vi "Zamojski_Target_C_1.vi"() -> ()   [LabVIEW 2020]
uses:
  <vilib>/Platform/TimedLoop/XDataNode/timing_clust.ctl
  <vilib>/Platform/TimedLoop/XDataNode/nitl_modes.ctl
  <vilib>/Platform/TimedLoop/XDataNode/wakeup.ctl
  <vilib>/platform/TimedLoop/XDataNode/XDataNode.xnode
  <vilib>/Platform/TimedLoop/XDataNode/XDNodeRunTimeDep.lvlib
panel:
  out "timed out?":bool
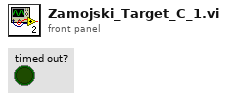
[diagram p1: front panel]
types:
  T1 = typedef "XDNodeRunTimeDep.lvlib/timing_clust.ctl" = cluster{"Expected End [f-1]":u64, "Actual End [f-1]":u64, "Finished Late? [f-1]":bool, "Expected End [i-1]":u64, "Actual End [i-1]":u64, "Finished Late? [i-1]":bool, "Expected Start [i]":u64, "Actual Start [i]":u64, "Expected Start [f]":u64, "Actual Start [f]":u64, "Source Name":string, "Structure Name":string, "Period":i64, "Deadline":i64, "Offset":i64, "Start":i64, "Priority":i32, "Timeout":i32, "Mode":T2, "Wakeup Reason":T3, "Error":errorcluster, "Source Type":string, "Secondary Source Type":string, "Global End Time":u64, "Global Start Time":u64, "Frame Duration":u64, "Iteration Duration":u64, "Assigned CPU":i32, "I/O Scan Engine Mode":u32}
  T2 = typedef "XDNodeRunTimeDep.lvlib/nitl_modes.ctl" = enum32{"No Change", "Process missed periods, maintain original phase", "Discard missed periods, maintain original phase", "Process missed periods, ignore original phase", "Discard missed periods, ignore original phase"}
  T3 = typedef "XDNodeRunTimeDep.lvlib/wakeup.ctl" = enum32{"Normal", "Aborted", "Asynchronous wakeup", "Timing source error", "Timed loop error", "Timeout"}
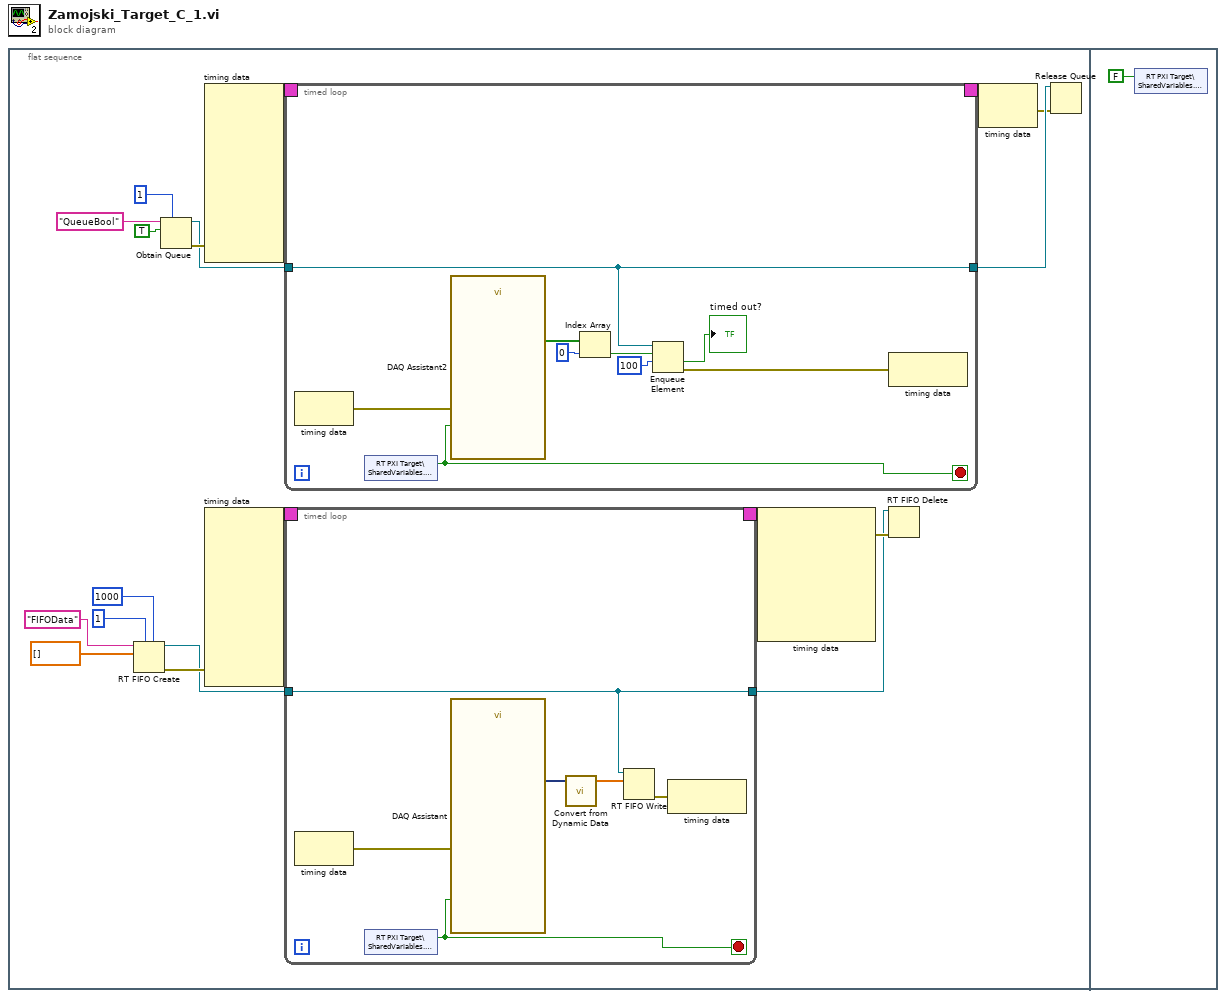
[diagram p0: block diagram]
diagram:
  n1 = flat-sequence {
    frame #0 {
      n2 = RT FIFO Create(0:"FIFOData" ("name (unnamed)"), 1:dbl[] [], 4:u32 1 ("size (10)"), 6:u32 1000 ("elements in array (1)")) -> (8:w11:refnum<k33>, 11:w15:errorcluster)  [unwired: 4 in, 1 out]
      n3 = Obtain Queue(max queue size (-1, unlimited)=1, name (unnamed)="QueueBool", element data type=TRUE) -> (queue out=w4:refnum<queue>, error out=w8:errorcluster)  [unwired: 2 in, 1 out]
      n4 = node-c288(w8) -> (w17:T1)  [unwired: 9 in]
      n5 = node-c288(w15) -> (w19:T1)  [unwired: 9 in]
      n6 = timed-loop {
        timing: w17 -> [_]
        timing-out: [_] -> w16
        tunnel: w4 -> [w21]
        tunnel: [w21] -> w3
        stop <- w24 stop-if-true
        n7 = node-c288() -> (w25:errorcluster)  [unwired: 1 in]
        n8 = shared-variable "RT PXI Target\\SharedVariables.lvlib\\STOP"() -> (w24:bool)  [unwired: 1 in, 1 out]
        n9 = call "DAQ Assistant2"("error in"=w25, "stop (T)"=w24) -> ("data"=w26:bool[])  [unwired: 15 in, 2 out]
        n10 = Index Array(array=w26, index=0) -> (element=w27:bool)
        n11 = Enqueue Element(queue=w21, element=w27, timeout in ms (-1)=100) -> (timed out?=→"timed out?":bool, error out=w23:errorcluster)  [unwired: 1 in, 1 out]
        n12 = node-c288(w23) -> ()  [unwired: 1 out]
      }
      n13 = timed-loop {
        timing: w19 -> [_]
        timing-out: [_] -> w18
        tunnel: w11 -> [w43]
        tunnel: [w43] -> w9
        stop <- w42 stop-if-true
        n14 = node-c288() -> (w40:errorcluster)  [unwired: 1 in]
        n15 = shared-variable "RT PXI Target\\SharedVariables.lvlib\\STOP"() -> (w42:bool)  [unwired: 1 in, 1 out]
        n16 = call "DAQ Assistant"("error in"=w40, "stop (T)"=w42) -> ("data"=w44:dynamicdata)  [unwired: 15 in, 2 out]
        n17 = call "Convert from Dynamic Data"("Dynamic Data Type"=w44) -> ("Array"=w39:dbl[])  [unwired: 3 in]
        n18 = RT FIFO Write(0:w43, 1:w39) -> (11:w41:errorcluster)  [unwired: 3 in, 3 out]
        n19 = node-c288(w41) -> ()  [unwired: 1 out]
      }
      n20 = node-c288(w18) -> (w10:errorcluster)  [unwired: 6 out]
      n21 = RT FIFO Delete(0:w9, 3:w10) -> ()  [unwired: 1 in, 1 out]
      n22 = node-c288(w16) -> (w2:errorcluster)
      n23 = Release Queue(queue=w3, error in (no error)=w2) -> ()  [unwired: 1 in, 3 out]
    }
    frame #1 {
      n24 = shared-variable "RT PXI Target\\SharedVariables.lvlib\\STOP"(FALSE ("STOP")) -> ()  [unwired: 1 in, 1 out]
    }
  }
